vi "putHardpointData.vi"(8 "error in (no error)":errorcluster, 10 "TelemetryHardpointData":T1, 11 "M1M3SAL in":refnum<class "M1M3SAL.lvclass">) -> (0 "error out":errorcluster, 3 "M1M3SAL out":refnum<class "M1M3SAL.lvclass">)   [LabVIEW 2016, in "M1M3SupportCommunicator.lvlib" / "M1M3SAL.lvclass"]
uses:
  M1M3SAL.lvclass
  DataTypes/Topics/TelemetryHardpointData.ctl
  DataTypes/Topics/Parts/Timestamp.ctl
  DataTypes/MessageHeader.ctl
  DataTypes/MessageTypes.ctl
  DataTypes/MessageTopics.ctl
  M1M3SAL.lvclass/M1M3SAL.ctl
  writeU8.vi
  writeI32.vi
  writeI16.vi
  writeSGL.vi
  writeBoolean.vi
  M1M3SupportCommunicator.lvlib
  DataTypes/Topics/M1M3SupportTopics.lvlib
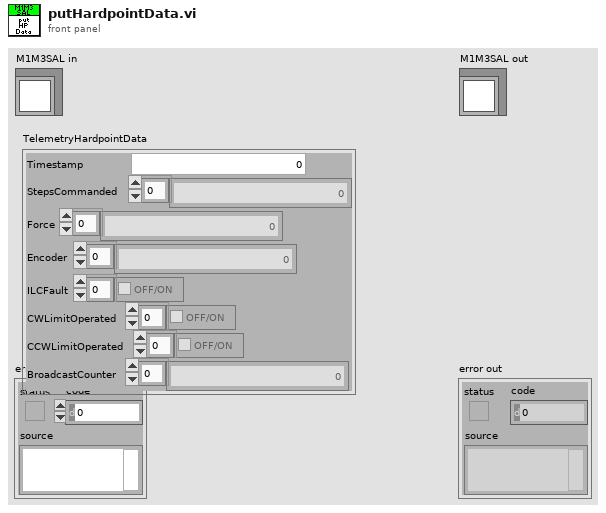
[diagram p1: front panel]
types:
  T1 = typedef "M1M3SupportTopics.lvlib/TelemetryHardpointData.ctl" = cluster{"Timestamp":T2, "StepsCommanded":i16[], "Force":sgl[], "Encoder":i32[], "ILCFault":bool[], "CWLimitOperated":bool[], "CCWLimitOperated":bool[], "BroadcastCounter":u8[]}
  T2 = typedef "M1M3SupportTopics.lvlib/Timestamp.ctl" = dbl
  T3 = typedef "M1M3SupportCommunicator.lvlib/MessageHeader.ctl" = cluster{"Type":T4, "Topic":T5, "Size":i32}
  T4 = typedef "M1M3SupportCommunicator.lvlib/MessageTypes.ctl" = enum8{"None", "PutSample", "GetNextSample", "LogEvent", "GetEvent", "IssueCommand", "CommandId", "WaitForCompletion", "AcceptCommand", "AckCommand"}
  T5 = typedef "M1M3SupportCommunicator.lvlib/MessageTopics.ctl" = enum8{"None", "ForceActuatorData", "MirrorForceData", "HardpointData", "AirData", "DynamicData", "FPGAData", "IMSData", "ForceActuatorStatus", "ElevationData", "HardpointStatus", "HardpointActuatorChase", "AirStatus", "ForceActuatorSafetyChecks", "ForceActuatorTest", "ActuatorBroadcastCounter", "StatusChecks", "CellChecks", "HardpointActuatorBreakaway", "RaiseMirrorComplete", "ILCCommunication", "ElevationAngleChecks", "DetailedState", "ServoLoops", "ForceActuatorInfo", "LowerMirrorComplete", "HardpointActuatorInfo", "SettingsApplied", "ErrorCode", "StartupChecks", "SummaryState", "SettingVersions", "ActuatorTestStatus", "AppliedSettingsMatchStart", "Enable", "EnterMaintenance", "Standby", "AbortLowerM1M3", "ApplyAberrationByForces", "ApplyAOSCorrectionByBendingModes", "ClearAOSCorrection", "Start", "RaiseM1M3", "TestForceActuator", "LowerM1M3", "ApplyAOSCorrectionByForces", "Disable", "ApplyAberationByBendingMode", "TestHardpoint", "ManipulateM1M3", "ClearAberration", "Exit", "TestAir", "AbortRaiseM1M3", "MoveHardpointActuators", "ExitMaintenance", "Shutdown"}
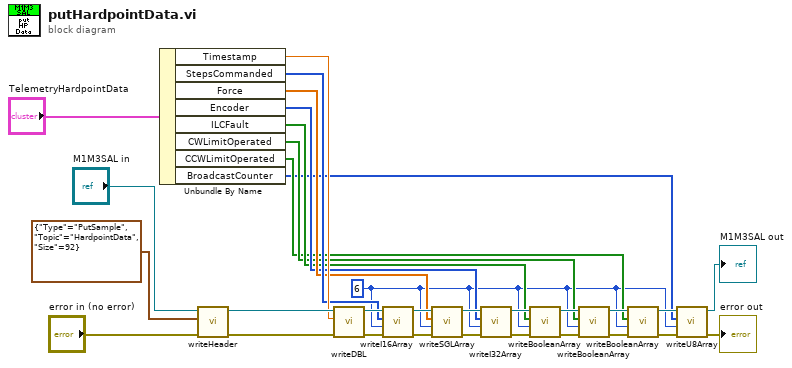
[diagram p0: block diagram]
diagram:
  w4 = 6 ("Length")
  n1 = Unbundle By Name("TelemetryHardpointData") -> ("Timestamp"=w14:T2, "StepsCommanded"=w13:i16[], "Force"=w12:sgl[], "Encoder"=w11:i32[], "ILCFault"=w10:bool[], "CWLimitOperated"=w9:bool[], "CCWLimitOperated"=w8:bool[], "BroadcastCounter"=w5:u8[])
  n2 = call "writeHeader.vi"("error in (no error)"="error in (no error)", "MessageHeader"=T3 {"Type"=enum."PutSample", "Topic"=enum."HardpointData", "Size"=92}, "M1M3SAL in"="M1M3SAL in") -> ("error out"=w19:errorcluster, "M1M3SAL out"=w24:refnum<class "M1M3SAL.lvclass">)  [unwired: 7 in]
  n3 = call "writeDBL.vi"("error in (no error)"=w19, "Input"=w14, "M1M3SAL in"=w24) -> ("error out"=w18:errorcluster, "M1M3SAL out"=w23:refnum<class "M1M3SAL.lvclass">)  [unwired: 7 in]
  n4 = call "writeI16Array.vi"("error in (no error)"=w18, "Length"=w4, "Input"=w13, "M1M3SAL in"=w23) -> ("error out"=w17:errorcluster, "M1M3SAL out"=w22:refnum<class "M1M3SAL.lvclass">)  [unwired: 6 in]
  n5 = call "writeSGLArray.vi"("error in (no error)"=w17, "Length"=w4, "Input"=w12, "M1M3SAL in"=w22) -> ("error out"=w16:errorcluster, "M1M3SAL out"=w21:refnum<class "M1M3SAL.lvclass">)  [unwired: 6 in]
  n6 = call "writeI32Array.vi"("error in (no error)"=w16, "Length"=w4, "Input"=w11, "M1M3SAL in"=w21) -> ("error out"=w15:errorcluster, "M1M3SAL out"=w20:refnum<class "M1M3SAL.lvclass">)  [unwired: 6 in]
  n7 = call "writeBooleanArray.vi"("error in (no error)"=w15, "Length"=w4, "Input"=w10, "M1M3SAL in"=w20) -> ("error out"=w28:errorcluster, "M1M3SAL out"=w27:refnum<class "M1M3SAL.lvclass">)  [unwired: 6 in]
  n8 = call "writeBooleanArray.vi"("error in (no error)"=w28, "Length"=w4, "Input"=w9, "M1M3SAL in"=w27) -> ("error out"=w26:errorcluster, "M1M3SAL out"=w25:refnum<class "M1M3SAL.lvclass">)  [unwired: 6 in]
  n9 = call "writeBooleanArray.vi"("error in (no error)"=w26, "Length"=w4, "Input"=w8, "M1M3SAL in"=w25) -> ("error out"=w6:errorcluster, "M1M3SAL out"=w7:refnum<class "M1M3SAL.lvclass">)  [unwired: 6 in]
  n10 = call "writeU8Array.vi"("error in (no error)"=w6, "Length"=w4, "Input"=w5, "M1M3SAL in"=w7) -> ("error out"=→"error out":errorcluster, "M1M3SAL out"=→"M1M3SAL out":refnum<class "M1M3SAL.lvclass">)  [unwired: 6 in]
